vi "Module Name or ID.vi"(10 "Module ID in":i32, 11 "Connection Name":string) -> (2 "Module ID out":i32)   [LabVIEW 2017, in "SSH.lvlib"]
doc: "Selects between using a module name or clone ID - if the module name is an empty string, it will get the use the module ID. If the module name has a value, it will look up the module ID in the FGV"
uses:
  SSH.lvlib
  Module Names FGV Actions.ctl
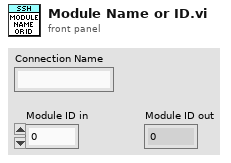
[diagram p1: front panel]
types:
  T1 = typedef "Module Names FGV Actions.ctl" = enum16{"Get", "Set"}
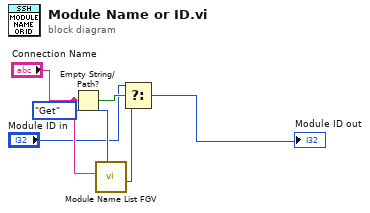
[diagram p0: block diagram]
diagram:
  n1 = Empty String/Path?(string/path="Connection Name") -> (empty?=w2:bool)
  n2 = call "Module Name List FGV.vi"("Action"=Module_Names_FGV_Actions."Get", "Name"="Connection Name") -> ("Module ID out"=w5:i32)  [unwired: 9 in]
  n3 = Select(t="Module ID in", s=w2, f=w5) -> (s? t:f=→"Module ID out":i32)
